vi "Get_ref_inst_value.vi"(0 "Ref Instrument type":T1, 2 "ADAM Channel Name":string, 7 "Index in":i32, 13 "Start time":dbl format="%.2f") -> (4 "Ref Value":dbl format="%.2f", 10 "Index out":i32)   [LabVIEW 2011]
uses:
  Controls/Ref_Inst_type.ctl
  Globals/Meas_global.vi
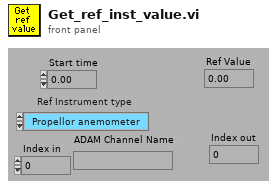
[diagram p1: front panel]
types:
  T1 = typedef "Ref_Inst_type.ctl" = enum16{"Propellor anemometer", "Pressure Transducer", "Raw voltage", "Pitot-static tube", "Preston tube", "Generic Linear", "Generic Polynomial", "Thermocouple", "LDA", "Enter Value", "ADAM Channel"}
  T2 = typedef "Analysis_info_cluster.ctl" = cluster{"Colour":u32, "Inst type":T3, "Inst name":string, "Symbol":string, "Code name":string, "Extra Info":string, "Inst Array":T4, "Index":i32, "Voltage Index":i32, "Extra Titles":string[], "Extra Values":string[], "Eng Values":dbl[], "Time (ms)":dbl[], "TT / Voltage":dbl[], "U":dbl, "u^2":dbl, "u^3":dbl, "u^4":dbl, "Skew_u":dbl, "Kurt_u":dbl, "Sd Error in Mean":dbl, "% u'/U":dbl, "X":dbl, "Y":dbl, "Z":dbl, "Spectra":T5, "Autocorrelation":T5, "Timescale integral to 25%":dbl, "Sd Error in Variance":dbl, "Calib File":path, "Calib Constants":dbl[], "Histogram":T5, "Output Position":bool, "Full Stats":bool}
  T3 = typedef "Inst_type.ctl" = enum16{"Propeller anemometer", "Raw voltage", "Pressure Transducer", "Pitot-static tube", "Preston tube", "Hot wire", "Cross wire 1", "Cross wire 2", "Generic Linear", "Generic Polynomial", "Generic BackPoly", "Fast FID", "Thermocouple", "Cold wire", "Pulsed Wire", "LDA Vel", "LDA Tran time", "LDA Arr time"}
  T4 = typedef "Instrument_Array.ctl" = enum16{"PWA", "LDA", "Analogue"}
  T5 = typedef "XY_Plot_Cluster.ctl" = cluster{"First Name":string, "Second Name":string, "X axis name":string, "Y axis name":string, "X array":dbl[], "Y array":dbl[]}
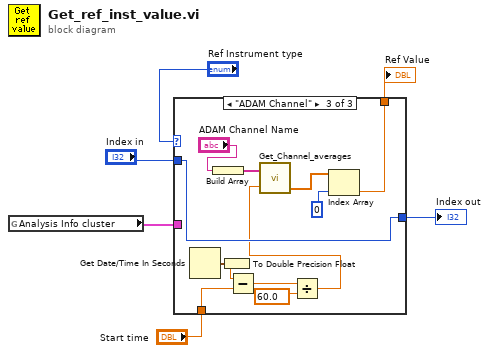
[diagram p0: block diagram]
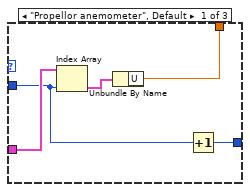
[diagram p2: hidden frame]
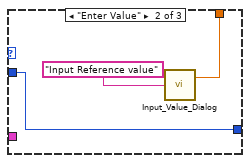
[diagram p3: hidden frame]
diagram:
  n1 = global read "Meas_global.vi" "Analysis Info cluster"() -> (w1:T2[])
  n2 = case shown="\"ADAM Channel\"" "Ref Instrument type" {
    tunnel: [w9 w14 w17] -> w4
    tunnel: "Index in" -> [w8 w12 w26]
    tunnel: "Start time" -> [_ _ w23]
    tunnel: w1 -> [w11 _ _]
    tunnel: [w7 w12 w26] -> w3
    frame "Propellor anemometer", Default {
      n3 = Index Array(array=w11, index=w8) -> (element=w10:T2)
      n4 = Unbundle By Name(w10) -> ("U"=w9:dbl)
      n5 = Increment(x=w8) -> (x+1=w7:i32)
    }
    frame "Enter Value" {
      n6 = call "Input_Value_Dialog.vi"("Message to user"="Input Reference value") -> ("Value received"=w14:dbl)  [unwired: 1 out]
    }
    frame "ADAM Channel" {
      n7 = Get Date/Time In Seconds() -> (seconds since 1Jan1904=w16:timestamp)
      n8 = Build Array("ADAM Channel Name") -> (w25:string[])
      n9 = To Double Precision Float(number=w16) -> (double precision float=w24:dbl)
      n10 = Subtract(x=w24, y=w23) -> (x-y=w22:dbl)
      n11 = Divide(x=w22, y=60.0) -> (x/y=w20:dbl)
      n12 = call "Get_Channel_averages.vi"("Desired Ch Names"=w25, "Averaging time (mins)"=w20) -> ("number"=w19:dbl[])  [unwired: 1 in, 2 out]
      n13 = Index Array(array=w19, index=0 ("Index")) -> (element=w17:dbl)
    }
  }
  "Index out" <- w3
  "Ref Value" <- w4
